vi "Get SMO PGSQL Log Paths.vi"(5 "getAll Cluster":variant, 7 "Paths":string="llab_038:d000(TEST_TABLE--Temperature(Kelvin))\nllab_038:d002(TEST_TABLE--voltage 2(volts))\nllab_038:b000(TEST_TABLE--ON?())\nllab_038:v001(TEST_TABLE--sample())", 8 "error in (no error)":errorcluster, 11 "Inst.MOTOR in":refnum<class "Inst.MOTOR.lvclass">) -> (0 "error out":errorcluster, 2 "Paths":string, 3 "Inst.MOTOR out":refnum<class "Inst.MOTOR.lvclass">)   [LabVIEW 2019, in "Inst.MOTOR.lvclass"]
uses:
  Inst.MOTOR.lvclass
  Typedefs/Inst.MOTOR.getAll--Cluster.ctl
  <userlib>/LevyLab/Instrument Framework/Instrument Types/VSource/Instrument.VSource.lvclass
  <userlib>/LevyLab/LV-Data/LV-Data.PG/LV-Data.PGSQL.lvclass
  <userlib>/LevyLab/LV-Data/LV-Data.PG/API/Write Variable (one-row).vi
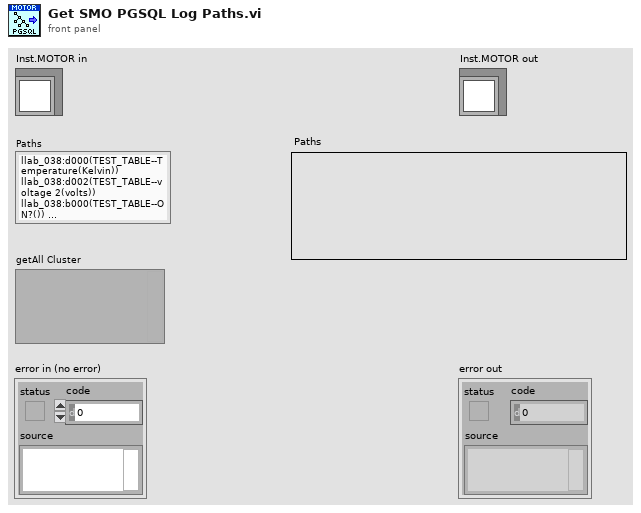
[diagram p1: front panel]
types:
  T1 = typedef "Inst.MOTOR.lvclass/Inst.MOTOR.getAll--Cluster.ctl" = cluster{"Response":string, "Forward":bool, "Stop Motor":bool, "Encoder Position":string}
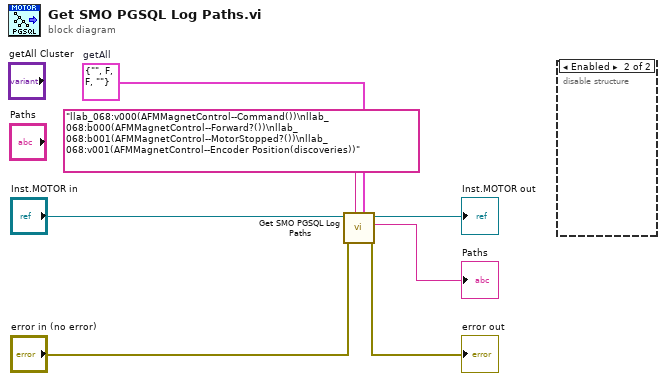
[diagram p0: block diagram]
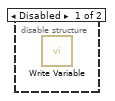
[diagram p2: hidden frame]
diagram:
  w1 = T1 {"Response"="", "Forward"=FALSE, "Stop Motor"=FALSE, "Encoder Position"=""}  # getAll
  n1 = call-parent "Get SMO PGSQL Log Paths.vi"("getAll Cluster"=w1, "Default Paths"="llab_068:v000(AFMMagnetControl--Command())\nllab_068:b000(AFMMagnetControl--Forward?())\nllab_068:b001(AFMMagnetControl--MotorStopped?())\nllab_068:v001(AFMMagnetControl--Encoder Position(discoveries))" ("Paths"), "error in (no error)"="error in (no error)", "Instrument in"="Inst.MOTOR in") -> ("error out"=→"error out":errorcluster, "Paths"=→"Paths":string, "Instrument out"=→"Inst.MOTOR out":refnum<class "Inst.MOTOR.lvclass">)  [unwired: 5 in]
  n2 = disable-structure shown="Enabled" {
    frame Disabled {
      n3 = call-poly <userlib>:"Write Variable.vi"() -> ()  [unwired: 8 in, 4 out]
    }
    frame Enabled {
    }
  }
